vi "Find Disconnection Route.vi"(8 "error in (no error)":errorcluster, 9 "channel 2":string, 10 "channel 1":string, 11 "Route Manager in":refnum<class "Route Manager.lvclass">) -> (0 "error out":errorcluster, 1 "relays to close":string[](array[string]), 2 "relays to open":string[](array[string]))   [LabVIEW 2015, in "Route Manager.lvclass"]
uses:
  Route Manager.lvclass
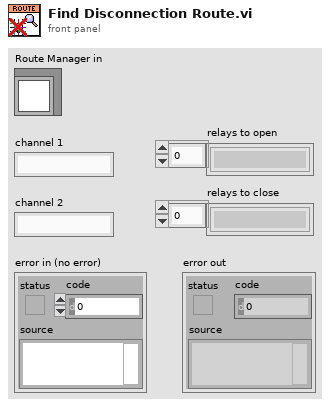
[diagram p1: front panel]
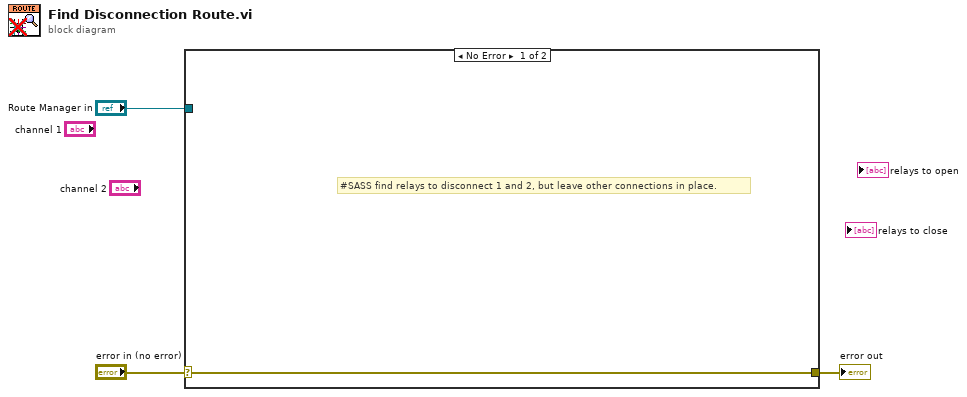
[diagram p0: block diagram]
diagram:
  n1 = case shown="No Error" "error in (no error)" {
    selector: "error in (no error)" -> [w4 w5]
    tunnel: [w4 w5] -> w2
    tunnel: "Route Manager in" -> [_ _]
    frame No Error {
      # "#SASS find relays to disconnect 1 and 2, but leave other connections in place."
    }
    frame Error {
    }
  }
  "error out" <- w2
